vi "cfgPFC_packet_encoder.vi"(11 "Control settings":T1) -> (3 "concatenated string":string)   [LabVIEW 2015, in "Hardware.lvlib"]
uses:
  Hardware.lvlib
  Settings/PFC Control settings.ctl
  PI Compensator.ctl
  Settings/Settings.lvlib
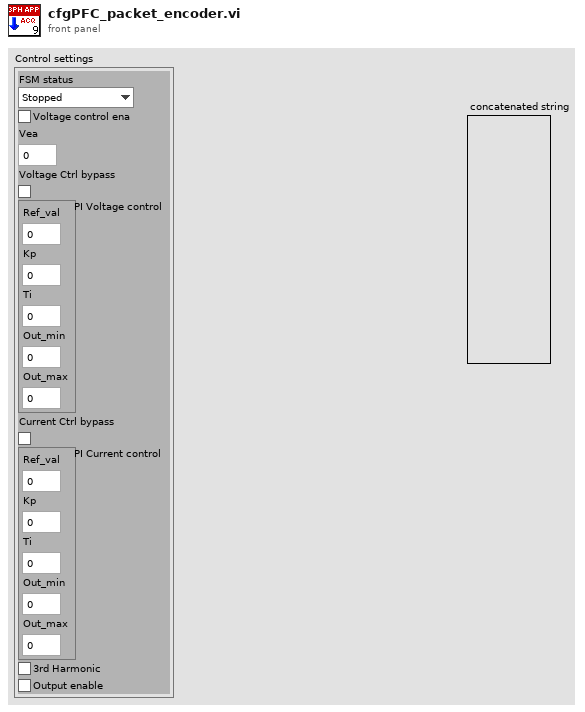
[diagram p1: front panel]
types:
  T1 = typedef "Settings.lvlib/PFC Control settings.ctl" = cluster{"FSM status":enum8{"Stopped", "Running"}, "Voltage control ena":bool, "Vea":sgl, "Voltage Ctrl bypass":bool, "PI Voltage control":T2, "Current Ctrl bypass":bool, "PI Current control":T2, "3rd Harmonic":bool, "Output enable":bool}
  T2 = typedef "Settings.lvlib/PI Compensator.ctl" = cluster{"Ref_val":sgl, "Kp":sgl, "Ti":sgl, "Out_min":sgl, "Out_max":sgl}
  T3 = enum16{"big-endian, network order", "native, host order", "little-endian"}
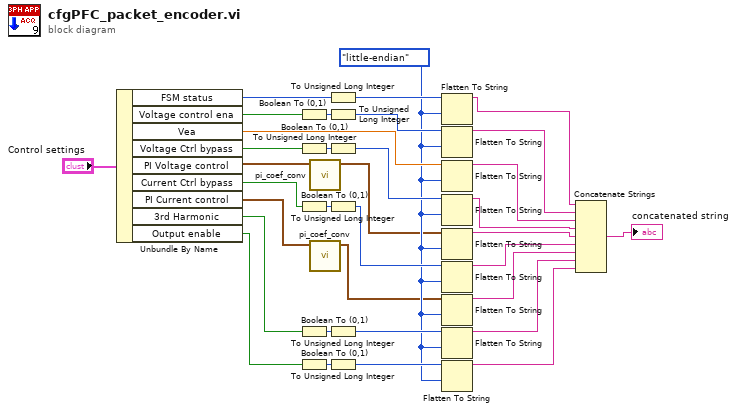
[diagram p0: block diagram]
diagram:
  w7 = T3."little-endian" ("byte order (0:big-endian, network order)")
  n1 = Unbundle By Name("Control settings") -> ("FSM status"=w33:enum8{"Stopped", "Running"}, "Voltage control ena"=w31:bool, "Vea"=w32:sgl, "Voltage Ctrl bypass"=w10:bool, "PI Voltage control"=w3:T2, "Current Ctrl bypass"=w15:bool, "PI Current control"=w1:T2, "3rd Harmonic"=w17:bool, "Output enable"=w18:bool)
  n2 = Boolean To (0,1)(Boolean=w31) -> (0, 1=w28:i16)
  n3 = Boolean To (0,1)(Boolean=w10) -> (0, 1=w9:i16)
  n4 = Boolean To (0,1)(Boolean=w15) -> (0, 1=w11:i16)
  n5 = Boolean To (0,1)(Boolean=w17) -> (0, 1=w13:i16)
  n6 = Boolean To (0,1)(Boolean=w18) -> (0, 1=w12:i16)
  n7 = call "pi_coef_conv.vi"("PI Control input"=w3) -> ("PI Control output"=w2:T2)  [unwired: 10 in]
  n8 = call "pi_coef_conv.vi"("PI Control input"=w1) -> ("PI Control output"=w4:T2)  [unwired: 10 in]
  n9 = To Unsigned Long Integer(number=w33) -> (unsigned 32bit integer=w29:u32)
  n10 = To Unsigned Long Integer(number=w28) -> (unsigned 32bit integer=w27:u32)
  n11 = To Unsigned Long Integer(number=w9) -> (unsigned 32bit integer=w8:u32)
  n12 = To Unsigned Long Integer(number=w11) -> (unsigned 32bit integer=w14:u32)
  n13 = To Unsigned Long Integer(number=w13) -> (unsigned 32bit integer=w16:u32)
  n14 = To Unsigned Long Integer(number=w12) -> (unsigned 32bit integer=w19:u32)
  n15 = Flatten To String(anything=w29, byte order (0:big-endian, network order)=w7) -> (data string=w30:string)  [unwired: 2 in, 2 out]
  n16 = Flatten To String(anything=w27, byte order (0:big-endian, network order)=w7) -> (data string=w26:string)  [unwired: 2 in, 2 out]
  n17 = Flatten To String(anything=w32, byte order (0:big-endian, network order)=w7) -> (data string=w24:string)  [unwired: 2 in, 2 out]
  n18 = Flatten To String(anything=w8, byte order (0:big-endian, network order)=w7) -> (data string=w5:string)  [unwired: 2 in, 2 out]
  n19 = Flatten To String(anything=w2, byte order (0:big-endian, network order)=w7) -> (data string=w6:string)  [unwired: 2 in, 2 out]
  n20 = Flatten To String(anything=w14, byte order (0:big-endian, network order)=w7) -> (data string=w23:string)  [unwired: 2 in, 2 out]
  n21 = Flatten To String(anything=w4, byte order (0:big-endian, network order)=w7) -> (data string=w22:string)  [unwired: 2 in, 2 out]
  n22 = Flatten To String(anything=w16, byte order (0:big-endian, network order)=w7) -> (data string=w21:string)  [unwired: 2 in, 2 out]
  n23 = Flatten To String(anything=w19, byte order (0:big-endian, network order)=w7) -> (data string=w20:string)  [unwired: 2 in, 2 out]
  n24 = Concatenate Strings(w30, w26, w24, w5, w6, w23, w22, w21, w20) -> (→"concatenated string":string)
